vi "Write Encoded UTF-8 String.vi"(9 "Encoded UTF-8 String":T1) -> (1 "UTF-8 String":refnum<class "UTF-8 String.lvclass">)   [LabVIEW 2020, in "G-Unicode.lvlib" / "UTF-8 String.lvclass"]
doc: "Set the UTF-8 string with an already encoded LabVIEW string.\n\nThe LabVIEW string is assumed to be UTF-8 encoded. Use <b>New UTF-8 String.vi</b> for converting a LabVIEW string to a UTF-8 string."
uses:
  UTF-8 String.lvclass
  Encoded UTF-8 String.ctl
  UTF-8 String.lvclass/UTF-8 String.ctl
  G-Unicode.lvlib
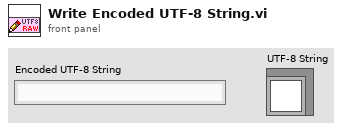
[diagram p1: front panel]
types:
  T1 = typedef "G-Unicode.lvlib/Encoded UTF-8 String.ctl" = string
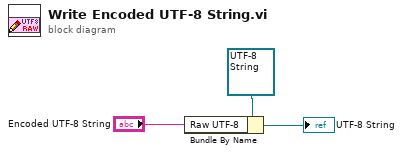
[diagram p0: block diagram]
diagram:
  n1 = Bundle By Name(cluster=refnum<class "UTF-8 String.lvclass"> refnum ("G-Unicode.lvlib:UTF-8.lvclass"), "Raw UTF-8"="Encoded UTF-8 String") -> (→"UTF-8 String":refnum<class "UTF-8 String.lvclass">)
